vi "Query Safety Interlock.vi"(8 "error in (no error)":errorcluster, 11 "VISA resource name":refnum<visa-resource-name>) -> (0 "error out":errorcluster, 2 "Safety Interlock":i32, 3 "VISA resource name out":refnum<visa-resource-name>)   [LabVIEW 2020, in "Keithley 6517.lvlib"]
doc: "Checks if the safety interlock cable is connected to the Model 6517B.\nThe response message is interpreted as follows:\n1 = Interlock cable connected to the 6517B and fixture, fixture lid or interlock switch is closed.\n0 = Interlock cable connected to 6517B but not connected to fixture, or interlock cable connected to 6517B but fixture lid is open, or no interlock cable connected.\n\nIf the interlock cable is not connected, the Model 6517B cannot determine the state of the test fixture lid (open or closed) or read the test fixture switch settings. The voltage source is then disabled."
uses:
  <instrlib>/Keithley 6517/Keithley 6517.lvlib
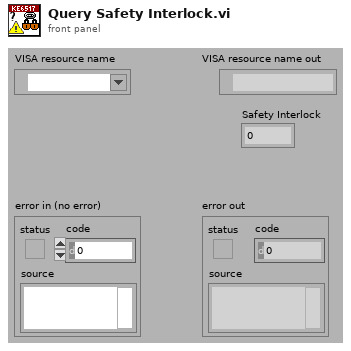
[diagram p1: front panel]
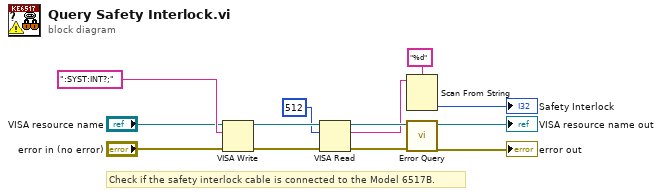
[diagram p0: block diagram]
diagram:
  # "Check if the safety interlock cable is connected to the Model 6517B."
  n1 = VISA Write(VISA resource name="VISA resource name", write buffer=":SYST:INT?;", error in (no error)="error in (no error)") -> (VISA resource name out=w8:refnum<visa-resource-name>, error out=w7:errorcluster)  [unwired: 1 out]
  n2 = VISA Read(VISA resource name=w8, byte count=u32 512, error in (no error)=w7) -> (VISA resource name out=w6:refnum<visa-resource-name>, read buffer=w3:string, error out=w5:errorcluster)  [unwired: 1 out]
  n3 = Scan From String(format string="%d", input string=w3) -> (output 1=→"Safety Interlock":i32)  [unwired: 3 in, 3 out]
  n4 = call <instrlib>:"Error Query.vi"("error in (no error)"=w5, "VISA resource name"=w6) -> ("error out"=→"error out":errorcluster, "VISA resource name out"=→"VISA resource name out":refnum<visa-resource-name>)  [unwired: 6 in, 2 out]
